vi "Examen.vi"() -> ()   [LabVIEW 2020]
uses:
  <vilib>/numeric/Random Number (Range) I64.vi
  <vilib>/numeric/sub_Random U32.vi
panel:
  out "Cantidad de muestras":dbl
  out "Tabla":string[][](array[string])
  out "Señal sin filtrar":dbl
  out "Rango":bool
  out "Histéresis":bool
  out "Waveform Chart":cluster{dbl, dbl}(graph)
  out "Señal de EMA":dbl
  out "Número random":u64
  in  "Botón de paro":bool
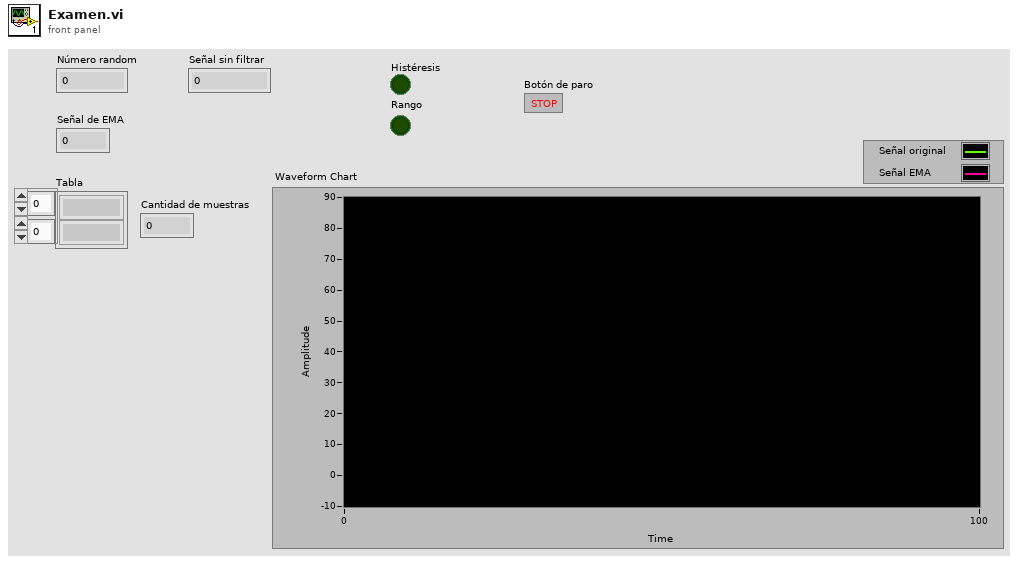
[diagram p1: front panel]
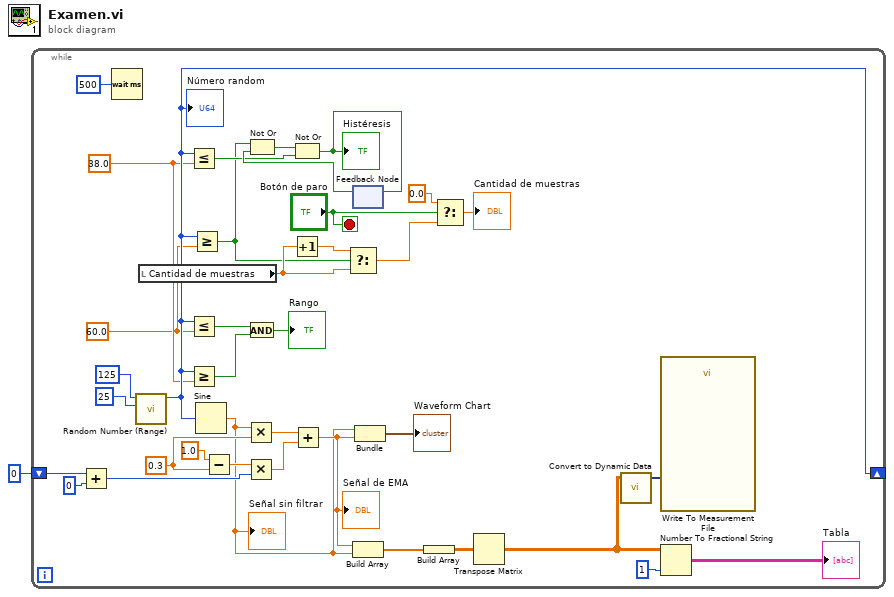
[diagram p0: block diagram]
diagram:
  n1 = while {
    shift-right: [w20] -> _
    shift-left: 0 -> [w35]
    stop <- "Botón de paro" stop-if-true
    w2 = 60.0 ("Lim_max")
    w3 = 38.0 ("Lim_min")
    w30 = 0.3 ("y")
    n2 = Add(x=w35, y=i64 0) -> (x+y=w33:i64)
    n3 = Wait (ms)(milliseconds to wait=u32 500) -> ()  [unwired: 1 out]
    n4 = call-poly <vilib>:"Random Number (Range).vi"("lower bound (-100)"=25, "upper bound (100)"=125) -> ("number"=w20:i64)  [unwired: 9 in]
    "Número random" <- w20
    n5 = local read "Cantidad de muestras"() -> (w10:dbl)
    n6 = Less Or Equal?(x=w20, y=w3) -> (x <= y?=w25:bool)
    n7 = Less Or Equal?(x=w20, y=w2) -> (x <= y?=w21:bool)
    n8 = Greater Or Equal?(x=w20, y=w3) -> (x >= y?=w22:bool)
    n9 = Greater Or Equal?(x=w20, y=w2) -> (x >= y?=w8:bool)
    n10 = Sine(x=w20) -> (sin(x)=w12:dbl)
    "Señal sin filtrar" <- w12
    n11 = Subtract(x=1.0, y=w30) -> (x-y=w32:dbl)
    n12 = Multiply(x=w12, y=w30) -> (x*y=w31:dbl)
    n13 = Multiply(x=w32, y=w33) -> (x*y=w28:dbl)
    n14 = And(x=w21, y=w22) -> (x .and. y?=→"Rango":bool)
    n15 = Increment(x=w10) -> (x+1=w9:dbl)
    n16 = Add(x=w31, y=w28) -> (x+y=w14:dbl)
    "Señal de EMA" <- w14
    n17 = Select(t=w9, s=w8, f=w10) -> (s? t:f=w6:dbl)
    n18 = feedback #1() -> (w26:bool)  [unwired: 1 in]
    n19 = Not Or(1:w26, 2:w8) -> (0:w27:bool)
    n20 = Not Or(1:w25, 2:w27) -> (0:w24:bool)
    "Histéresis" <- w24
    n21 = feedback-in #1(w24) -> ()
    n22 = Build Array(w14, w12) -> (w13:dbl[])
    n23 = Bundle(w12, w14) -> (→"Waveform Chart":cluster{dbl, dbl})  [unwired: 1 in]
    n24 = Build Array(w13) -> (w11:dbl[][])
    n25 = Select(t=0.0, s="Botón de paro", f=w6) -> (s? t:f=→"Cantidad de muestras":dbl)
    n26 = Transpose Matrix(1:w11) -> (0:w16:dbl[][])
    n27 = call "Convert to Dynamic Data"("2D Array"=w16) -> ("Dynamic Data Type"=w19:dynamicdata)  [unwired: 3 in]
    n28 = call "Write To Measurement File"("Signals"=w19) -> ()  [unwired: 16 in, 3 out]
    n29 = Number To Fractional String(number=w16, precision (6)=i16 1) -> (F-format string=→"Tabla":string[][])  [unwired: 2 in]
  }
